vi "Gas_Status_panel.vi"(7 "Ch names":string[](array[string])) -> (1 "Trace Gas":string, 2 "Trace Hi-Tec Range":string, 10 "Gas Remaining":string[][](table), 12 "Carrier Gas 1":string, 13 "Carrier Gas 2":string, 14 "Carrier 1 Hi-Tec Range":string)   [LabVIEW 2022 SP3]
uses:
  Anemometry/Anemometry Sub Vis/Globals/Gas_management_global.vi
  Anemometry/Anemometry Sub Vis/Globals/Preference_global.vi
panel:
  out "Atmos Pres (mbars)":string
  # "Carrier Gas"
  # "Trace Gas"
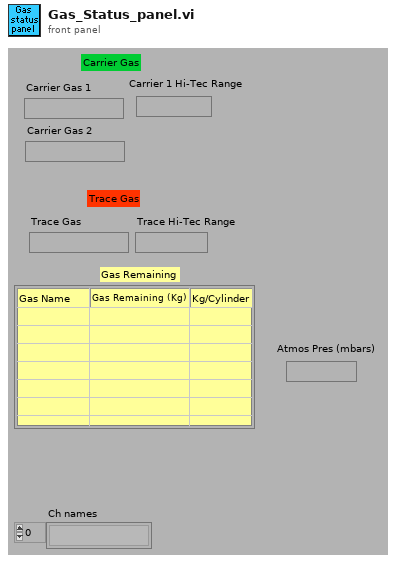
[diagram p1: front panel]
types:
  T1 = enum16{"Gas Remaining", "Trace Gas", "Carrier Gas", "Atmospheric Pressure"}
  T2 = typedef "Ch_description_ADAM.ctl" = cluster{"Ch Name":string, "Type":T3, "Function":T4, "Ch State":T5, "Calibration type":T6, "A":dbl, "B":dbl, "C":dbl, "D":dbl, "Comments":string, "Address":T7, "String":string, "Duty":u16}
  T3 = typedef "Module_type_ADAM.ctl" = string
  T4 = typedef "Function_ADAM.ctl" = enum16{"Analogue Input", "Digital Input", "Event counter", "Event rate", "Analogue Output", "Digital Output", "Relay Output"}
  T5 = typedef "Channel_State.ctl" = enum16{"On", "Off", "Always On", "Always Off"}
  T6 = typedef "Calib_type_ADAM.ctl" = string
  T7 = typedef "Address.ctl" = cluster{"Main":i32, "Ch.":i32, "Sub":i32, "Port Name":string}
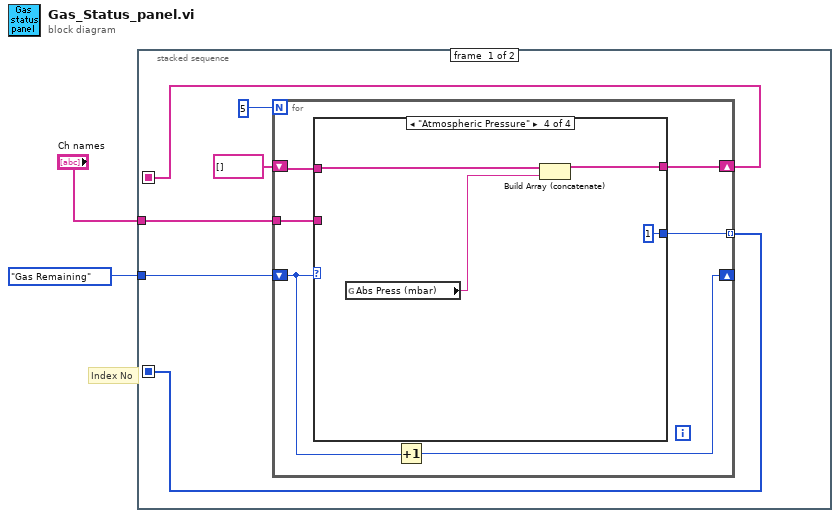
[diagram p0: block diagram]
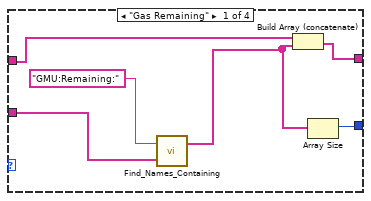
[diagram p2: hidden frame]
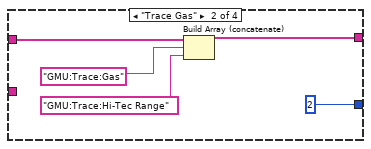
[diagram p3: hidden frame]
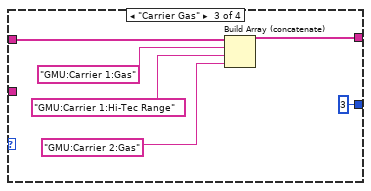
[diagram p4: hidden frame]
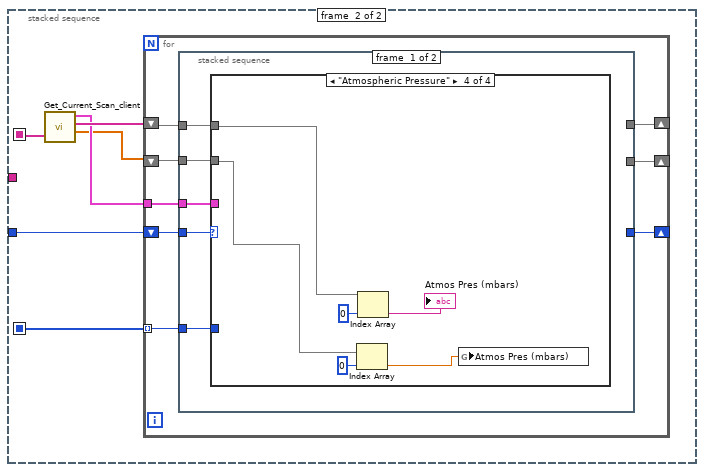
[diagram p5: hidden frame]
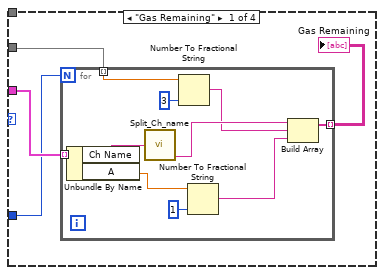
[diagram p6: hidden frame]
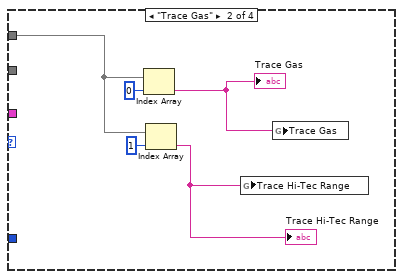
[diagram p7: hidden frame]
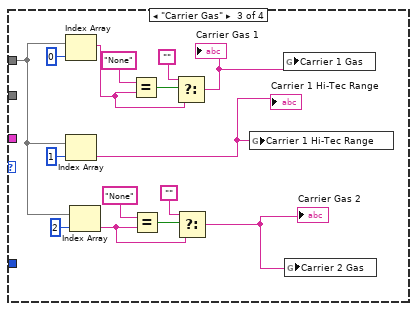
[diagram p8: hidden frame]
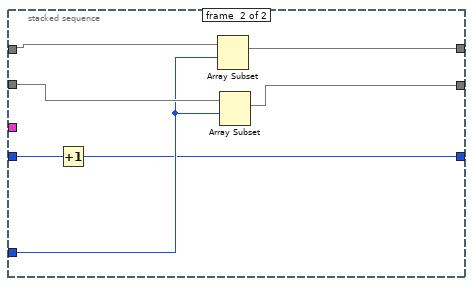
[diagram p9: hidden frame]
diagram:
  # "Index No"
  n1 = stacked-sequence {
    seq-local: [w6 _] -> [_ w40]
    seq-local: [w4 _] -> [_ w37]
    tunnel: T1."Gas Remaining" -> [w8 w41]
    tunnel: "Ch names" -> [w5 _]
    frame #0 {
      n2 = for {
        N: 5 -> [_]
        shift-right: [w13] -> _
        shift-left: w8 -> [w14]
        shift-right: [w11] -> w6
        shift-left: string[] [] -> [w12]
        tunnel: w5 -> [w10]
        tunnel: [w9] -> w4 mode=indexing
        n3 = case shown="\"Atmospheric Pressure\"" w14 {
          tunnel: w12 -> [w19 w25 w31 w35]
          tunnel: [w18 w24 w30 w34] -> w11
          tunnel: w10 -> [w20 _ _ _]
          tunnel: [w16 2 3 1] -> w9
          frame "Gas Remaining" {
            n4 = call "Find_Names_Containing.vi"("Ch names"=w20, "String to match"="GMU:Remaining:") -> ("Matched Names"=w17:string[])  [unwired: 1 out]
            n5 = Build Array (concatenate)(w19, w17) -> (w18:string[])
            n6 = Array Size(array=w17) -> (size(s)=w16:i32)
          }
          frame "Trace Gas" {
            n7 = Build Array (concatenate)(w25, "GMU:Trace:Gas", "GMU:Trace:Hi-Tec Range") -> (w24:string[])
          }
          frame "Carrier Gas" {
            n8 = Build Array (concatenate)(w31, "GMU:Carrier 1:Gas", "GMU:Carrier 1:Hi-Tec Range", "GMU:Carrier 2:Gas") -> (w30:string[])
          }
          frame "Atmospheric Pressure" {
            n9 = global read "Preference_global.vi" "Abs Press (mbar)"() -> (w32:string)
            n10 = Build Array (concatenate)(w35, w32) -> (w34:string[])
          }
        }
        n11 = Increment(x=w14) -> (x+1=w13:T1)
      }
    }
    frame #1 {
      n12 = call "Get_Current_Scan_client.vi"("multipleChannels"=w40) -> ("Ch Description Array"=w38:T2[], "String values"=w39:string[], "Numerical Values"=w36:dbl[])  [unwired: 1 in, 1 out]
      n13 = for {
        shift-right: [w42] -> _
        shift-left: w41 -> [w47]
        shift-right: [w48] -> _
        shift-left: w39 -> [w49]
        tunnel: w38 -> [w46]
        tunnel: w37 -> [w45] mode=indexing
        shift-right: [w43] -> _
        shift-left: w36 -> [w44]
        n14 = stacked-sequence {
          tunnel: w49 -> [w54 w101]
          tunnel: [_ w98] -> w48
          tunnel: w47 -> [w53 w96]
          tunnel: w46 -> [w52 _]
          tunnel: w45 -> [w51 w99]
          tunnel: w44 -> [w50 w100]
          tunnel: [_ w97] -> w43
          tunnel: [_ w95] -> w42
          frame #0 {
            n15 = case shown="\"Atmospheric Pressure\"" w53 {
              tunnel: w54 -> [_ w69 w84 w90]
              tunnel: w52 -> [w58 _ _ _]
              tunnel: w51 -> [w56 _ _ _]
              tunnel: w50 -> [w55 _ _ w89]
              frame "Gas Remaining" {
                n16 = for {
                  N: w56 -> [_]
                  tunnel: w58 -> [w68] mode=indexing
                  tunnel: [w62] -> w57 mode=indexing
                  tunnel: w55 -> [w60] mode=indexing
                  n17 = Unbundle By Name(w68) -> ("Ch Name"=w67:string, "A"=w65:dbl)
                  n18 = call "Split_Ch_name.vi"("Ch name"=w67) -> ("Low level"=w64:string)  [unwired: 2 out]
                  n19 = Number To Fractional String(number=w60, precision (6)=i16 3) -> (F-format string=w59:string)  [unwired: 2 out]
                  n20 = Number To Fractional String(number=w65, precision (6)=i16 1) -> (F-format string=w63:string)  [unwired: 2 out]
                  n21 = Build Array(w64, w59, w63) -> (w62:string[])
                }
                "Gas Remaining" <- w57
              }
              frame "Trace Gas" {
                n22 = Index Array(array=w69, index=0) -> (element=w71:string)
                "Trace Gas" <- w71
                n23 = Index Array(array=w69, index=1) -> (element=w70:string)
                "Trace Hi-Tec Range" <- w70
                n24 = global write "Gas_management_global.vi" "Trace Hi-Tec Range"(w70) -> ()
                n25 = global write "Gas_management_global.vi" "Trace Gas"(w71) -> ()
              }
              frame "Carrier Gas" {
                n26 = Index Array(array=w84, index=0) -> (element=w75:string)
                n27 = Index Array(array=w84, index=1) -> (element=w86:string)
                "Carrier 1 Hi-Tec Range" <- w86
                n28 = Index Array(array=w84, index=2) -> (element=w81:string)
                n29 = Equal?(x="None" ("y"), y=w75) -> (x = y?=w76:bool)
                n30 = Equal?(x="None" ("y"), y=w81) -> (x = y?=w83:bool)
                n31 = Select(t="", s=w76, f=w75) -> (s? t:f=w74:string)
                "Carrier Gas 1" <- w74
                n32 = Select(t="", s=w83, f=w81) -> (s? t:f=w79:string)
                "Carrier Gas 2" <- w79
                n33 = global write "Gas_management_global.vi" "Carrier 1 Hi-Tec Range"(w86) -> ()
                n34 = global write "Gas_management_global.vi" "Carrier 1 Gas"(w74) -> ()
                n35 = global write "Gas_management_global.vi" "Carrier 2 Gas"(w79) -> ()
              }
              frame "Atmospheric Pressure" {
                n36 = Index Array(array=w89, index=0) -> (element=w91:dbl)
                n37 = Index Array(array=w90, index=0) -> (element=→"Atmos Pres (mbars)":string)
                n38 = global write "Gas_management_global.vi" "Atmos Pres (mbars)"(w91) -> ()
              }
            }
          }
          frame #1 {
            n39 = Increment(x=w96) -> (x+1=w95:T1)
            n40 = Array Subset(array=w101, index=w99) -> (w98:string[])  [unwired: 1 in]
            n41 = Array Subset(array=w100, index=w99) -> (w97:dbl[])  [unwired: 1 in]
          }
        }
      }
    }
  }
